vi "Dashboard Main.vi"() -> ()   [LabVIEW 2017]
uses:
  <vilib>/event_ctls.llb/eventvkey.ctl
  <vilib>/Rock Robotics/WPI/Dashboard/WPI_DashboardLogging Global.vi
  <vilib>/Utility/miscctls.llb/LVRowAndColumnTypeDef.ctl
  <vilib>/Rock Robotics/Network Tables/NT Write Numeric Array.vi
  <vilib>/Rock Robotics/Network Tables/NT Read Numeric Array.vi
panel:
  in  "Camera Settings Right":T1={"Frame Rate"=30, "Compression"=30, "Size"=1, "DB Camera Config"=FALSE} {"Frame Rate" scale=1.0..30.0; "Compression" scale=100.0..-1.0; "Size" items=["640x480", "320x240", "160x120"]}
  in  "Camera Name Right":string(combo)="No Camera Selection"
  out "Camera Info":cluster{"Mbps LED":bool, "Mbps":dbl, "fps":dbl} {"fps" format="%#.1g"; "Mbps" format="%#.1g"}
  in  "Camera Settings":T1={"Frame Rate"=30, "Compression"=30, "Size"=1, "DB Camera Config"=FALSE} {"Frame Rate" scale=1.0..30.0; "Compression" scale=100.0..-1.0; "Size" items=["640x480", "320x240", "160x120"]}
  in  "TCP":refnum<k5>
  in  "Rec Mode":enum32{"Stop", "Record", "Playback"}(radio)
  out "Robot IP":string
  out "Image Message":string="Timeout in Camera Communications"
  in  "Dashboard Tab":T2(tab)
  in  "Select Auto":string(combo)="Select Autonomous ..."
  out "NT Connection":bool
  out "MotorChart R":cluster{"Numeric":dbl, "Numeric":dbl}(graph)
  out "MotorChart L":cluster{"Numeric":dbl, "Numeric":dbl}(graph)
  out "MotorSliders R":cluster{"MotorSlide1":dbl, "MotorSlide2":dbl} {"MotorSlide2" scale=-1.0..1.0 scale format="%#_2e"; "MotorSlide1" scale=-1.0..1.0 scale format="%#_2e"}
  out "MotorSliders L":cluster{"MotorSlide1":dbl, "MotorSlide2":dbl} {"MotorSlide2" scale=-1.0..1.0 scale format="%#_2e"; "MotorSlide1" scale=-1.0..1.0 scale format="%#_2e"}
  out "Gyro":dbl(knob) scale=0.0..360.0
  out "JS1 Z":dbl(slide) scale=-1.0..1.0 scale format="%#_2e"
  out "JS1 Graph":cluster{"X":dbl, "Y":dbl}[](graph)
  out "JS1 Buttons":T3
  out "JS2 Z":dbl(slide) scale=-1.0..1.0 scale format="%#_2e"
  out "JS2 Graph":cluster{"X":dbl, "Y":dbl}[](graph)
  out "JS2 Buttons":T3
  out "Mode":T4(ring)=enum."Auto Disabled"
  out "Camera Image Right":T5(plugin-control)
  out "Left Encoder":dbl
  out "Right Encoder":dbl
  in  "Teleop Controls":T6(tab)
  in  "Y Axis":T7
  in  "X Axis":T7
  in  "Forward Trim":T8={"Trim Max"=0.37, "Trim Min"=0.01, "Trim Deadzone"=0.1, "Trim LR"=TRUE}
  in  "Backward Trim":T8={"Trim Max"=0.5, "Trim Min"=0.05, "Trim Deadzone"=0.1, "Trim LR"=FALSE}
  in  "PID Tuning":enum32{"Drive with PID", "Turn by Angle"}(tab)
  in  "Drive with PID":T9={"Max Speed"=0.7, "P/I/D"=[1.0, 0.0, 0.01], "Min Speed"=0.4, "Accel Distance"=64.0}
  in  "Turn By Angle":T10={"P/I/D"=[0.25, 0.001, 0.0], "Turn Speed"=0.55, "Linearity"=0.6}
  in  "Autonomous Distances":T11(tab)
  in  "Station 1 Angle":dbl=60.0
  in  "Station 1":dbl[](array[numeric])=[97.0, 30.0, -30.0, 120.0]
  in  "Station 2":dbl[](array[numeric])=[82.0, -48.0, 48.0, 120.0]
  in  "Station 3 Angle":dbl=-60.0
  in  "Station 3":dbl[](array[numeric])=[96.0, 30.0, -30.0, 120.0]
  in  "Drive Forward":dbl[](array[numeric])=[82.0, 0.0, 0.0, 0.0]
  in  "Gear and B":dbl[](array[numeric])=[82.0, -48.0, 0.0, 0.0]
  in  "Test Slider":dbl(slide) scale=0.0..100.0 scale format="%#_3g"
  in  "On/Off":bool caption="Solenoid"
  in  "Test Name":u16(ring) items=["Select the test to run..."]
  in  "Test Tree":string(tree)
  in  "Motor":cluster{"Value":dbl, "Enable":bool} {"Value" scale=-1.0..1.0 scale format="%#_3g"}
  out "Progress":T12 {"Test Progress" scale=0.0..100.0}
  in  "Rev/Fwd":cluster{"Forward":bool, "Reverse":bool}
  in  "Test Ring":u16(ring) items=["Monochrome", "Color"]
  out "Cmd Status":string
  in  "Execute Command":bool
  in  "Command Params":string[][](table)
  in  "Command Selection":i32(listbox)
  in  "CheckList":i32(listbox)
  out "Tree":string(tree)
  out "Camera Image":T5(plugin-control)
  in  "Camera Name":string(combo)="No Camera Selection"
  out "Background":bool
  # "HW"
  # "HW"
  # "Joysticks"
  # "Drive Motors"
  # "Front"
  # "Right"
  # "Left"
  # "Back"
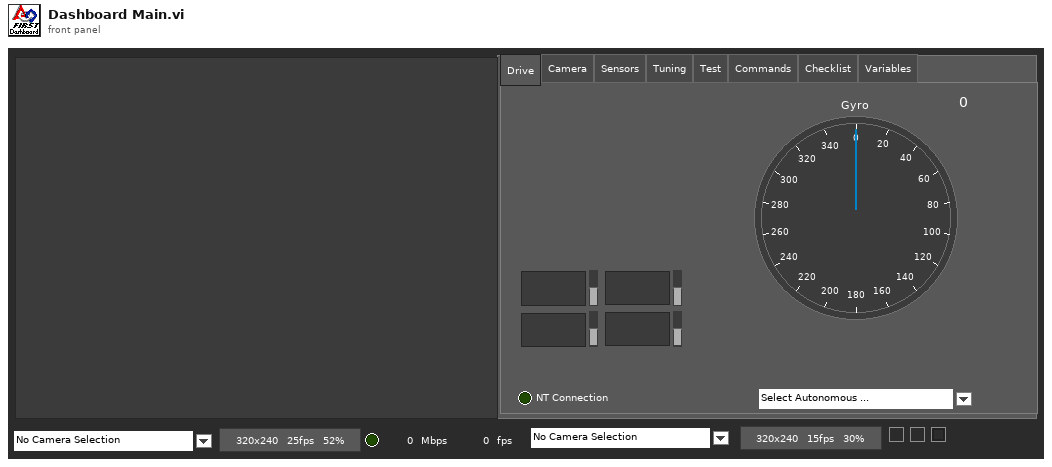
[diagram p1: front panel]
types:
  T1 = cluster{"Frame Rate":i32, "Compression":i32, "Size":u16, "DB Camera Config":bool}
  T2 = enum32{"Drive", "Camera", "Sensors", "Tuning", "Test", "Commands", "Checklist", "Variables"}
  T3 = cluster{bool, bool, bool, bool, bool, bool, bool, bool, bool, bool, bool, bool}
  T4 = enum8{"Tele-Op Disabled", "Tele-Op Enabled", "Auto Disabled", "Auto Enabled", "Test Disabled", "Test Enabled", "Disconnected", "No Code", "E-Stop"}
  T5 = typedef "IMAQ Image.ctl" = refnum<image>
  T6 = enum32{"Speed Sensitivity", "Turn Sensitivity", "Forward Trim", "Backwards Trim"}
  T7 = cluster{"Max Speed":dbl, "Min Speed":dbl, "Deadzone":dbl}
  T8 = cluster{"Trim Max":dbl, "Trim Min":dbl, "Trim Deadzone":dbl, "Trim LR":bool}
  T9 = cluster{"Max Speed":dbl, "P/I/D":dbl[], "Min Speed":dbl, "Accel Distance":dbl}
  T10 = cluster{"P/I/D":dbl[], "Turn Speed":dbl, "Linearity":dbl}
  T11 = enum32{"Station 1", "Station 2", "Station 3", "Drive Forward", "Gear and Back"}
  T12 = cluster{"Test Progress":u8, "Test Progress Text":string}
  T13 = typedef "Image Type" = u32
  T14 = cluster{"IDs":cluster{"RPC field ID":u16, "Unique ID":u16}, "String":string}
  T15 = enum32{"Drive", "Basic", "Custom", "Test", "Checklist", "Variables"}
  T16 = cluster{"Error Strings":string, "Disable Counts":cluster{u16, u16}, "Rail Faults":cluster{u16, u16, u16}, "Robot IP":string, "DB Mode":u8, "Event Info":cluster{"Name":string, "Type":u8, "Number":u16, "Replay":u8}}
  T17 = cluster{"Storage":cluster{"Disk Free":u64, "RAM Block":u32, "RAM free":u32}, "CPU Utilization":cluster{"CPU % ISR":sgl, "CPU % Time Crit":sgl, "CPU % Timed Str":sgl, "CPU % High":sgl, "CPU % Above":sgl, "CPU % Normal":sgl, "CPU % Low":sgl}, "CAN":cluster{"% Bus Utilization":sgl, "Bus Off Cnt":u32, "TX_FIFO Full Cnt":u32, "Receive Error Cnt":u8, "Transmit Error Cnt":u8}, "HID":cluster{"HID Outputs":u32, "Rumble Low":u16, "Rumble High":u16}[]}
  T18 = cluster{"Status bits":cluster{"Test Mode":bool, "Autonomous":bool, "Enabled":bool, "Code Start":bool, "Brownout":bool, "Reserved 2":bool, "Reserved 3":bool, "E-Stop":bool}, "Code Trace":cluster{"Disabled":bool, "TeleOp":bool, "Auto":bool, "Test":bool}, "Controller Type":enum16{"unknown", "cRIO", "roboRio"}, "Code?":enum16{"unknown", "noCode", "code"}, "Battery V":dbl}
  T19 = cluster{"Control Bits":cluster{"TestMode":bool, "Autonomous":bool, "Enabled":bool, "FMS Present":bool, bool, bool, bool, "E-Stop":bool}, "Team Station ":u8, "Countdown":sgl, "Joystick Values":cluster{"Axes":dbl[], "Buttons":bool[], "POVs":i16[]}[]}
  T20 = cluster{"Axes":dbl[], "Buttons":bool[], "POVs":i16[]}[]
  T21 = cluster{"Axes":dbl[], "Buttons":bool[], "POVs":i16[]}
  T22 = cluster{"Buttons[0]":bool, "Buttons[1]":bool, "Buttons[2]":bool, "Buttons[3]":bool, "Buttons[4]":bool, "Buttons[5]":bool, "Buttons[6]":bool, "Buttons[7]":bool, "Buttons[8]":bool, "Buttons[9]":bool, "Buttons[10]":bool, "Buttons[11]":bool}
  T23 = cluster{"Camera Image":refnum<vi>, "Dashboard Tab":refnum<vi>, "Background":refnum<vi>, "Rec Mode":refnum<vi>, "Test Slider":refnum<vi>, "On/Off ":refnum<vi>, "Test Ring":refnum<vi>, "Rev/Fwd":refnum<vi>, "Test Name":refnum<vi>, "Motor":refnum<vi>, "Progress":refnum<vi>, "CheckList":refnum<vi>, "Tree":refnum<vi>, "Test Tree":refnum<vi>, "Command Params":refnum<vi>, "Command Selection":refnum<vi>, "Execute Command":refnum<vi>, "Cmd Status":refnum<vi>, "Camera Settings":refnum<vi>, "Camera Name":refnum<vi>, "Camera Info":refnum<vi>, "Camera Settings Right":refnum<vi>, "Camera Name Right":refnum<vi>, "Camera Image Right":refnum<vi>}
  T24 = cluster{"Operation":enum16{"Update", "Clear"}, "Color Box":u32}[]
  T25 = typedef "eventvkey.ctl" = enum16{"ASCII", "Enter", "Return", "Shift", "Ctrl", "Alt", "Cmd", "Opt", "Caps", "NumLock", "Clear", "Break", "Up", "Down", "Left", "Right", "Insert", "Delete", "Home", "End", "PageUp", "PageDown", "Escape", "Help", "Pause", "ScrollLock", "F1", "F2", "F3", "F4", "F5", "F6", "F7", "F8", "F9", "F10", "F11", "F12", "F13", "F14", "F15", "F16", "F17", "F18", "F19", "F20", "F21", "F22", "F23", "F24", "Play", "VolumeUp", "VolumeDown", "Mute", "Two Byte Char"}
  T26 = cluster{"Image Size":bool, "Image Type":bool, "Pixel Value":bool, "ROI Information":bool, "Zoom Factor":bool}
  T27 = cluster{"Operation":enum16{"Update", "Clear"}, "Color Box":u32}
  T28 = typedef "LVRowAndColumnTypeDef.ctl" = cluster{"Row":i32, "Column":i32}
  T29 = cluster{"Shift":bool, "Ctrl":bool, "Alt":bool, "Cmd":bool, "Opt":bool}
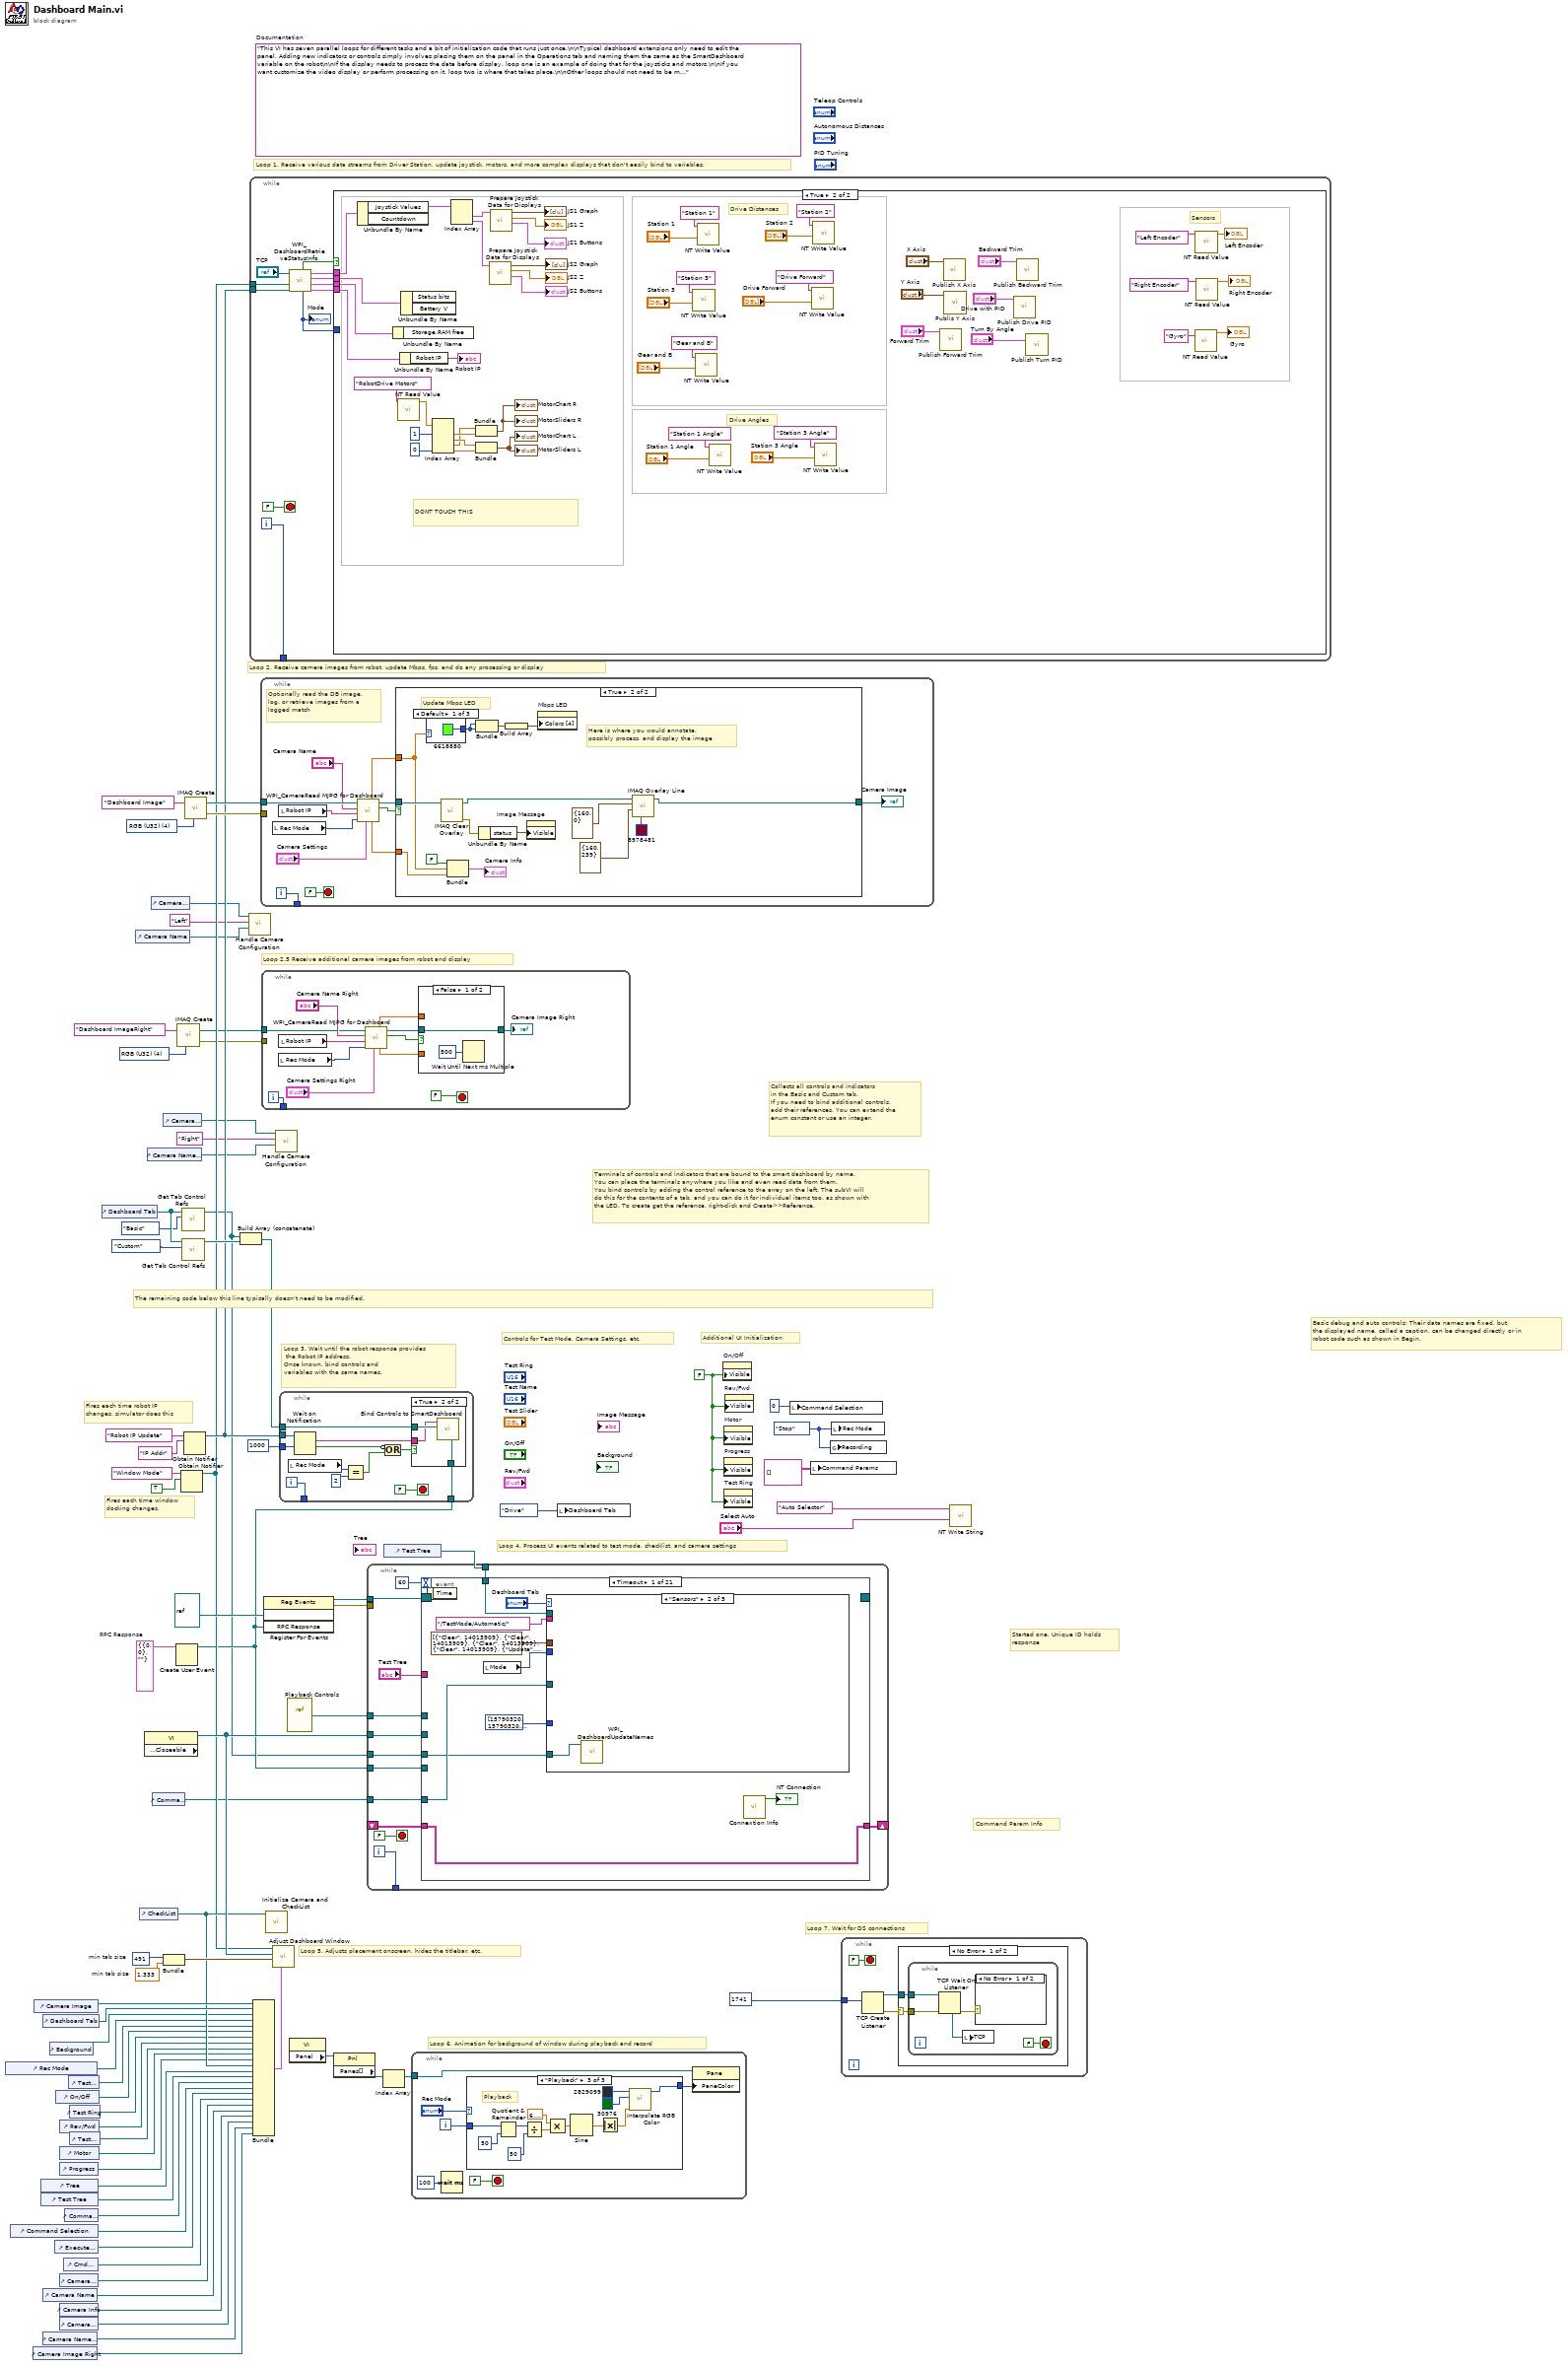
[diagram p0: block diagram]
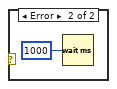
[diagram p3: hidden frame]
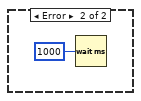
[diagram p4: hidden frame]
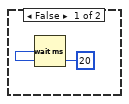
[diagram p5: hidden frame]
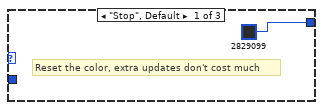
[diagram p6: hidden frame]
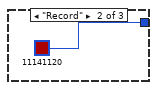
[diagram p7: hidden frame]
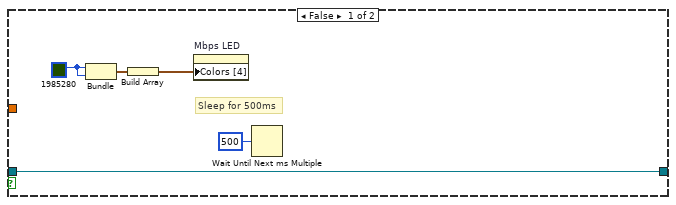
[diagram p9: hidden frame]
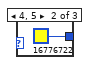
[diagram p10: hidden frame]
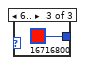
[diagram p11: hidden frame]
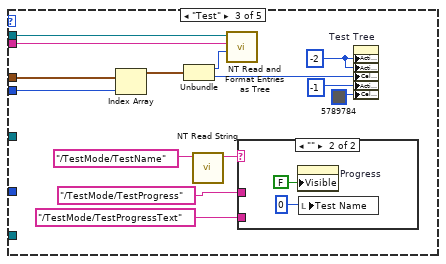
[diagram p13: hidden frame]
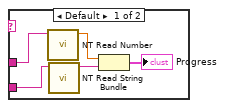
[diagram p14: hidden frame]
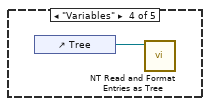
[diagram p15: hidden frame]
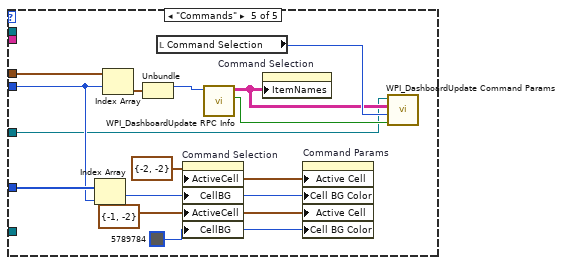
[diagram p16: hidden frame]
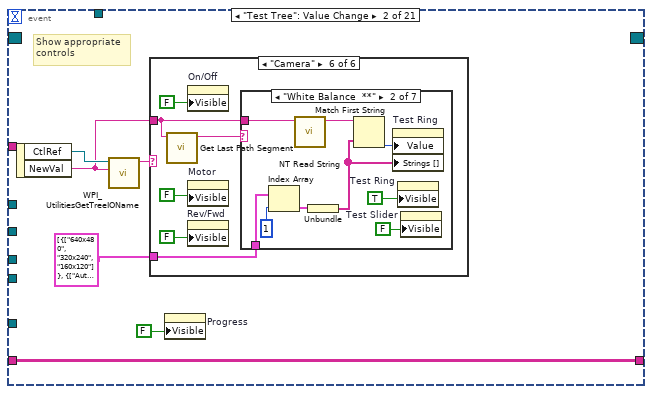
[diagram p17: hidden frame]
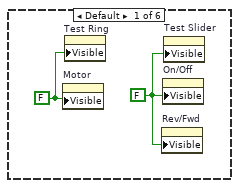
[diagram p18: hidden frame]
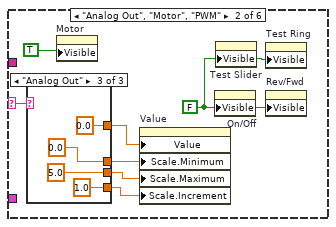
[diagram p19: hidden frame]
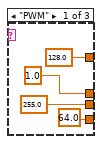
[diagram p20: hidden frame]
diagram:
  w11 = T13 4 items=["Grayscale (U8)", "Grayscale (I16)", "Grayscale (SGL)", "Complex (CSG)", "RGB (U32)", "HSL (U32)", "RGB (U64)"] ("Image Type")
  w27 = T14 {"IDs"={"RPC field ID"=0, "Unique ID"=0}, "String"=""}  # RPC Response
  w51 = 491  # min tab size
  w50 = 1.333  # min tab size
  w58 = enum32{"Stop", "Record", "Playback"}."Stop" ("Rec Mode")
  w34 = FALSE ("Visible")
  (unwired) "This VI has seven parallel loops for different tasks and a bit of initialization code that runs just once.\n\nTypical dashboard extensions only need to edit the panel. Adding new indicators or controls simply involves placing them on the panel in the Operations tab and naming them the same as the SmartDashboard variable on the robot\n\nIf the display needs to process the data before display, loop one is an example of doing that for the joysticks and motors.\n\nIf you want customize the video display or perform processing on it, loop two is where that takes place.\n\nOther loops should not need to be modified. They are pretty standard, and document the task they perform."  # Documentation
  w75 = T13 4 items=["Grayscale (U8)", "Grayscale (I16)", "Grayscale (SGL)", "Complex (CSG)", "RGB (U32)", "HSL (U32)", "RGB (U64)"] ("Image Type")
  # "Loop 2.5 Receive additional camera images from robot and display"
  # "Command Param Info"
  # "Started one, Unique ID holds\nresponse"
  # "Loop 7. Wait for DS connections"
  # "Basic debug and auto controls: Their data names are fixed, but\nthe displayed name, called a caption, can be changed directly or in\nrobot code such as shown in Begin."
  # "Controls for Test Mode, Camera Settings, etc."
  # "Additional UI Initialization"
  # "Loop 6. Animation for background of window during playback and record"
  # "Fires each time robot IP\nchanges, simulator does this"
  # "Fires each time window\ndocking changes."
  # "Collects all controls and indicators\nin the Basic and Custom tab.\nIf you need to bind additional controls,\nadd their references. You can extend the\nenum constant or use an integer."
  # "The remaining code below this line typically doesn't need to be modified."
  # "Loop 4. Process UI events related to test mode, checklist, and camera settings"
  # "Terminals of controls and indicators that are bound to the smart dashboard by name.\nYou can place the terminals anywhere you like and even read data from them.\nYou bind controls by adding the control reference to the array on the left. The subVI will\ndo this for the contents of a tab, and you can do it for individual items too, as shown with\nthe LED. To create get the reference, right-click and Create>>Reference."
  # "Loop 3. Wait until the robot response provides\n the Robot IP address.\nOnce known, bind controls and\nvariables with the same names."
  # "Loop 5. Adjusts placement onscreen, hides the titlebar, etc."
  # "Loop 1. Receive various data streams from Driver Station, update joystick, motors, and more complex displays that don't easily bind to variables."
  # "Loop 2. Receive camera images from robot, update Mbps, fps, and do any processing or display"
  n1 = control-ref of="Rec Mode"() -> (w40:refnum<vi>)
  n2 = control-ref of="Command Selection"() -> (w26:refnum<vi>)
  n3 = control-ref of="Camera Image Right"() -> (w2:refnum<vi>)
  n4 = control-ref of="Camera Image"() -> (w53:refnum<vi>)
  n5 = control-ref of="Tree"() -> (w44:refnum<vi>)
  n6 = control-ref of="Test Tree"() -> (w43:refnum<vi>)
  n7 = control-ref of="Dashboard Tab"() -> (w52:refnum<vi>)
  n8 = control-ref of="Camera Name"() -> (w17:refnum<vi>)
  n9 = control-ref of="Camera Name Right"() -> (w3:refnum<vi>)
  n10 = control-ref of="Background"() -> (w1:refnum<vi>)
  n11 = control-ref of="Execute Command"() -> (w28:refnum<vi>)
  n12 = control-ref of="On/Off"() -> (w38:refnum<vi>)
  n13 = control-ref of="Progress"() -> (w35:refnum<vi>)
  n14 = control-ref of="Camera Settings"() -> (w18:refnum<vi>)
  n15 = control-ref of="Camera Info"() -> (w16:refnum<vi>)
  n16 = control-ref of="Camera Settings Right"() -> (w4:refnum<vi>)
  n17 = control-ref of="Rev/Fwd"() -> (w36:refnum<vi>)
  n18 = control-ref of="Motor"() -> (w41:refnum<vi>)
  n19 = control-ref of="Cmd Status"() -> (w22:refnum<vi>)
  n20 = control-ref of="Command Params"() -> (w29:refnum<vi>)
  n21 = control-ref of="Test Slider"() -> (w39:refnum<vi>)
  n22 = control-ref of="Test Ring"() -> (w37:refnum<vi>)
  n23 = control-ref of="Test Name"() -> (w42:refnum<vi>)
  n24 = control-ref of="Dashboard Tab"() -> (w56:refnum<vi>)
  n25 = control-ref of="Camera Name"() -> (w19:refnum<vi>)
  n26 = control-ref of="CheckList"() -> (w45:refnum<vi>)
  n27 = property class="VI" props=["Front Panel.Closeable"]() -> (reference out=w57:refnum<vi>)  [unwired: 2 in, 2 out]
  n28 = control-ref of="Camera Name Right"() -> (w7:refnum<vi>)
  n29 = control-ref of="Camera Settings"() -> (w20:refnum<vi>)
  n30 = control-ref of="Command Params"() -> (w21:refnum<vi>)
  n31 = control-ref of="Camera Settings Right"() -> (w8:refnum<vi>)
  n32 = Bundle("min tab size"=w51, "min tab size"=w50) -> (w49:cluster{"min tab size":i32, "min tab size":dbl})  [unwired: 1 in]
  n33 = Create User Event(user event datatype=w27) -> (user event=w23:refnum<user-event>)  [unwired: 1 in, 1 out]
  n34 = call "IMAQ Create"("Image Name"="Dashboard ImageRight", "Image Type"=w11) -> ("New Image"=w10:T5, "error out"=w9:errorcluster)  [unwired: 2 in, 1 out]
  n35 = Obtain Notifier(name (unnamed)="Window Mode", notification data type=TRUE) -> (notifier out=w32:refnum<notifier>)  [unwired: 2 in, 2 out]
  n36 = call <vilib>:"Get Tab Control Refs.vi"("Page Index"=T15."Basic" ("Dashboard Tab"), "TabControl in"=w56) -> ("ControlsOnPage"=w15:refnum<vi>[])  [unwired: 9 in]
  n37 = call <vilib>:"Get Tab Control Refs.vi"("Page Index"=T15."Custom" ("Dashboard Tab"), "TabControl in"=w56) -> ("ControlsOnPage"=w55:refnum<vi>[])  [unwired: 9 in]
  n38 = Obtain Notifier(name (unnamed)="Robot IP Update", notification data type="IP Addr" ("name (unnamed)")) -> (notifier out=w33:refnum<notifier>)  [unwired: 2 in, 2 out]
  n39 = call "IMAQ Create"("Image Name"="Dashboard Image", "Image Type"=w75) -> ("New Image"=w73:T5, "error out"=w72:errorcluster)  [unwired: 2 in, 1 out]
  n40 = Build Array (concatenate)(w15, w55) -> (w54:refnum<vi>[])
  n41 = call "Handle Camera Configuration.vi"("CameraNameRef"=w19, "Camera File Name"="Left", "ClusterRef"=w20) -> ()  [unwired: 9 in]
  n42 = while {
    tunnel: [w85] -> _
    tunnel: w33 -> [w79]
    tunnel: w32 -> [w76]
    i -> [w85]
    stop <- FALSE stop-if-true
    n43 = call <vilib>:"WPI_DashboardRetrieveStatusInfo.vi"("Binding Refnum"=w79, "Window Mode Notifier"=w76, "TCP Cnx"="TCP") -> ("Power and Errors"=w80:T16, "Robot Metrics"=w83:T17, "Status Info"=w84:T18, "Control Info"=w81:T19, "Robot Mode"=w78:T4, "Process?"=w82:bool)  [unwired: 3 in]
    "Mode" <- w78
    n44 = case shown="True" w82 {
      tunnel: w84 -> [_ w137]
      tunnel: w83 -> [_ w136]
      tunnel: w81 -> [_ w135]
      tunnel: w80 -> [_ w134]
      tunnel: w78 -> [_ _]
      frame False {
        n45 = Wait (ms)(milliseconds to wait=u32 20) -> ()  [unwired: 1 out]
      }
      frame True {
        # "Drive Angles"
        # "Sensors"
        # "Drive Distances"
        # "DONT TOUCH THIS"
        n46 = Unbundle By Name(w135) -> ("Joystick Values"=w125:T20)  [unwired: 1 out]
        n47 = Unbundle By Name(w136) -> ()  [unwired: 1 out]
        n48 = call-poly <vilib>:"NT Read Value.vi"("Name"="RobotDrive Motors") -> ("Numeric Array"=w115:dbl[])  [unwired: 9 in, 1 out]
        n49 = Unbundle By Name(w134) -> ("Robot IP"=→"Robot IP":string)
        n50 = Unbundle By Name(w137) -> ()  [unwired: 2 out]
        n51 = Index Array(array=w115, index #1=1, index #4=0) -> (element #1=w129:dbl, element #2=w130:dbl, element #3=w128:dbl, element #4=w133:dbl)  [unwired: 2 in]
        n52 = Index Array(array=w125) -> (element #1=w124:T21, element #2=w120:T21)  [unwired: 2 in]
        n53 = Bundle("Numeric"=w128, "Numeric"=w129) -> (→"MotorChart R" →"MotorSliders R":cluster{"Numeric":dbl, "Numeric":dbl})  [unwired: 1 in]
        n54 = Bundle("Numeric"=w130, "Numeric"=w133) -> (→"MotorChart L" →"MotorSliders L":cluster{"Numeric":dbl, "Numeric":dbl})  [unwired: 1 in]
        n55 = call "Prepare Joystick Data for Displays.vi"("Joystick Values"=w120) -> ("Buttons"=→"JS2 Buttons":T22, "Z Axis"=→"JS2 Z":dbl, "Cartesian Data"=→"JS2 Graph":cluster{"X axis":dbl, "X axis":dbl}[])  [unwired: 8 in]
        n56 = call "Prepare Joystick Data for Displays.vi"("Joystick Values"=w124) -> ("Buttons"=→"JS1 Buttons":T22, "Z Axis"=→"JS1 Z":dbl, "Cartesian Data"=→"JS1 Graph":cluster{"X axis":dbl, "X axis":dbl}[])  [unwired: 8 in]
        n57 = call-poly <vilib>:"NT Write Value.vi"("Numeric Array"="Station 3", "Name"="Station 3") -> ()  [unwired: 9 in, 1 out]
        n58 = call-poly <vilib>:"NT Write Value.vi"("Numeric Array"="Gear and B", "Name"="Gear and B") -> ()  [unwired: 9 in, 1 out]
        n59 = call-poly <vilib>:"NT Write Value.vi"("Numeric Array"="Station 1", "Name"="Station 1") -> ()  [unwired: 9 in, 1 out]
        n60 = call-poly <vilib>:"NT Write Value.vi"("Numeric"="Station 1 Angle", "Name"="Station 1 Angle") -> ()  [unwired: 9 in, 1 out]
        n61 = call-poly <vilib>:"NT Write Value.vi"("Numeric Array"="Drive Forward", "Name"="Drive Forward") -> ()  [unwired: 9 in, 1 out]
        n62 = call-poly <vilib>:"NT Write Value.vi"("Numeric Array"="Station 2", "Name"="Station 2") -> ()  [unwired: 9 in, 1 out]
        n63 = call-poly <vilib>:"NT Write Value.vi"("Numeric"="Station 3 Angle", "Name"="Station 3 Angle") -> ()  [unwired: 9 in, 1 out]
        n64 = call "Publish Forward Trim.vi"("Forward Trim"="Forward Trim") -> ()  [unwired: 11 in]
        n65 = call "Publish X Axis.vi"("X Axis"="X Axis") -> ()  [unwired: 11 in]
        n66 = call "Publis Y Axis.vi"("Y Axis"="Y Axis") -> ()  [unwired: 11 in]
        n67 = call "Publish Drive PID.vi"("Drive with PID"="Drive with PID") -> ()  [unwired: 11 in]
        n68 = call "Publish Backward Trim.vi"("Backward Trim"="Backward Trim") -> ()  [unwired: 11 in]
        n69 = call "Publish Turn PID.vi"("Turn By Angle"="Turn By Angle") -> ()  [unwired: 11 in]
        n70 = call-poly <vilib>:"NT Read Value.vi"("Name"="Gyro") -> ("Numeric"=→"Gyro":dbl)  [unwired: 9 in, 1 out]
        n71 = call-poly <vilib>:"NT Read Value.vi"("Name"="Left Encoder") -> ("Numeric"=→"Left Encoder":dbl)  [unwired: 9 in, 1 out]
        n72 = call-poly <vilib>:"NT Read Value.vi"("Name"="Right Encoder") -> ("Numeric"=→"Right Encoder":dbl)  [unwired: 9 in, 1 out]
      }
    }
  }
  n73 = Bundle("Camera Image"=w53, "Dashboard Tab"=w52, "Background"=w1, "Rec Mode"=w40, "Test Slider"=w39, "On/Off"=w38, "Test Ring"=w37, "Rev/Fwd"=w36, "Test Name"=w42, "Motor"=w41, "Progress"=w35, "CheckList"=w45, "Tree"=w44, "Test Tree"=w43, "Command Params"=w29, "Command Selection"=w26, "Execute Command"=w28, "Cmd Status"=w22, "Camera Settings"=w18, "Camera Name"=w17, "Camera Info"=w16, "Camera Settings Right"=w4, "Camera Name Right"=w3, "Camera Image Right"=w2) -> (w46:T23)  [unwired: 1 in]
  n74 = while {
    tunnel: w73 -> [w147]
    tunnel: w72 -> [_]
    tunnel: [w148] -> _
    i -> [w148]
    stop <- FALSE stop-if-true
    # "Optionally read the DB image,\nlog, or retrieve images from a\nlogged match"
    n75 = local read "Rec Mode"() -> (w143:enum32{"Stop", "Record", "Playback"})
    n76 = local read "Robot IP"() -> (w142:string)
    n77 = call <vilib>:"WPI_CameraRead MJPG for Dashboard.vi"("Camera Settings"="Camera Settings", "Rec Mode"=w143, "NT Connection"=w142, "Capture Info"="Camera Name", "Refnum in"=w147) -> ("Active"=w145:bool, "Refnum out"=w146:T5, "FPS"=w144:dbl, "Bandwidth (Mbps)"=w141:dbl)  [unwired: 3 in]
    n78 = case shown="True" w145 {
      tunnel: w146 -> [w150 w165]
      tunnel: w141 -> [_ w162]
      tunnel: w144 -> [_ w163]
      tunnel: [w150 w158] -> w138
      frame False {
        w152 = u32 1985280 ("Color Box")
        # "Sleep for 500ms"
        n79 = Bundle("Color Box"=w152, "Color Box"=w152) -> (w153:cluster{"Color Box":u32, "Color Box":u32})  [unwired: 1 out]
        n80 = Build Array(w153) -> (w151:cluster{"Color Box":u32, "Color Box":u32}[])
        n81 = property on="Mbps LED" class="Bool (strict)"("Colors [4]"=w151) -> ()  [unwired: 2 in, 2 out]
        n82 = Wait Until Next ms Multiple(millisecond multiple=u32 500) -> ()  [unwired: 1 out]
      }
      frame True {
        # "Here is where you would annotate,\npossibly process, and display the image"
        # "Update Mbps LED"
        n83 = case shown="Default" w162 {
          tunnel: [u32 6618880 ("Color Box") u32 16776722 ("Color Box") u32 16716800 ("Color Box")] -> w166
          frame Default {
          }
          frame 4, 5 {
          }
          frame 6.. {
          }
        }
        n84 = call "IMAQ Clear Overlay"("Image"=w165) -> ("error out"=w168:errorcluster, "Image Out"=w159:T5)  [unwired: 2 in, 7 out]
        n85 = Bundle(FALSE, "Bandwidth (Mbps)"=w162, "FPS"=w163) -> (→"Camera Info":cluster{bool, "Bandwidth (Mbps)":dbl, "FPS":dbl})  [unwired: 1 in]
        n86 = Bundle("Color Box"=w166, "Color Box"=w166) -> (w167:cluster{"Color Box":u32, "Color Box":u32})  [unwired: 1 out]
        n87 = Unbundle By Name(w168) -> ("status"=w169:bool)
        n88 = Build Array(w167) -> (w164:cluster{"Color Box":u32, "Color Box":u32}[])
        n89 = property on="Image Message" class="Str"("Visible"=w169) -> ()  [unwired: 2 in, 2 out]
        n90 = property on="Mbps LED" class="Bool (strict)"("Colors [4]"=w164) -> ()  [unwired: 2 in, 2 out]
        n91 = call "IMAQ Overlay Line"("Color"=u32 8978481, "End Point"=cluster{"X":i32, "Y":i32} {"X"=160, "Y"=239}, "Start Point"=cluster{"X":i32, "Y":i32} {"X"=160, "Y"=0}, "Image"=w159) -> ("Image Out"=w158:T5)  [unwired: 6 in, 1 out]
      }
    }
    "Camera Image" <- w138
  }
  n92 = while {
    tunnel: w10 -> [w183]
    tunnel: w9 -> [_]
    tunnel: [w177] -> _
    i -> [w177]
    stop <- FALSE stop-if-true
    n93 = local read "Rec Mode"() -> (w181:enum32{"Stop", "Record", "Playback"})
    n94 = local read "Robot IP"() -> (w182:string)
    n95 = call <vilib>:"WPI_CameraRead MJPG for Dashboard.vi"("Camera Settings"="Camera Settings Right", "Rec Mode"=w181, "NT Connection"=w182, "Capture Info"="Camera Name Right", "Refnum in"=w183) -> ("Active"=w176:bool, "Refnum out"=w179:T5, "FPS"=w174:dbl, "Bandwidth (Mbps)"=w175:dbl)  [unwired: 3 in]
    n96 = case shown="False" w176 {
      tunnel: w179 -> [w185 w187]
      tunnel: w175 -> [_ _]
      tunnel: w174 -> [_ _]
      tunnel: [w185 w187] -> w173
      frame False {
        n97 = Wait Until Next ms Multiple(millisecond multiple=u32 500) -> ()  [unwired: 1 out]
      }
      frame True {
      }
    }
    "Camera Image Right" <- w173
  }
  n98 = register-events(refnum<vi> refnum, w23) -> (reference out=w62:refnum<event-registration>, error out=w61:errorcluster)  [unwired: 2 in]
  n99 = call "Initialize Camera and CheckList.vi"("ListBox in"=w45) -> ()  [unwired: 11 in]
  n100 = call "Adjust Dashboard Window.vi"("Sizing Refnums"=w46, "Size Constraints"=w49, "VI"=w57, "WIn Mode"=w32) -> ()  [unwired: 8 in]
  n101 = call "Handle Camera Configuration.vi"("CameraNameRef"=w7, "Camera File Name"="Right", "ClusterRef"=w8) -> ()  [unwired: 9 in]
  n102 = while {
    tunnel: w54 -> [w199]
    tunnel: w33 -> [w197]
    tunnel: [w195] -> _
    tunnel: u32 1000 ("milliseconds to wait") -> [w194]
    tunnel: w23 -> [w188]
    i -> [w195]
    stop <- FALSE stop-if-true
    n103 = local read "Rec Mode"() -> (w190:enum32{"Stop", "Record", "Playback"})
    n104 = Wait on Notification(notifier=w197, timeout in ms (-1)=w194) -> (notification=w196:string, timed out?=w192:bool)  [unwired: 2 in, 2 out]
    n105 = Equal?(x=w190, y=u16 2 ("Rec Mode")) -> (x = y?=w191:bool)
    n106 = Compound Arithmetic op=OR(invert w192, w191) -> (w193:bool)
    n107 = case shown="True" w193 {
      tunnel: w199 -> [_ w202]
      tunnel: w196 -> [_ w201]
      tunnel: w188 -> [_ w200]
      frame False {
      }
      frame True {
        n108 = call <vilib>:"Bind Controls to SmartDashboard.vi"("RPC ref"=w200, "Bound Control Refs"=w202, "Server IP Address"=w201) -> ()  [unwired: 9 in]
      }
    }
  }
  n109 = vi-ref "Playback Controls.vi"() -> (w63:refnum<vi>)
  n110 = property class="VI"() -> ("Panel"=w65:refnum<vi>)  [unwired: 2 in, 2 out]
  n111 = property class="Pnl"(reference=w65) -> ("Panes[]"=w66:refnum<vi>[])  [unwired: 1 in, 2 out]
  n112 = Index Array(array=w66) -> (element=w64:refnum<vi>)  [unwired: 1 in]
  n113 = control-ref of="Test Tree"() -> (w67:refnum<vi>)
  n114 = while {
    tunnel: [w212] -> _
    tunnel: w67 -> [w211]
    tunnel: w63 -> [w210]
    tunnel: w62 -> [w209]
    tunnel: w61 -> [_]
    tunnel: w57 -> [w208]
    tunnel: w23 -> [w207]
    tunnel: w21 -> [w206]
    shift-right: [w205] -> _
    shift-left: _ -> [w204]
    tunnel: w15 -> [w203]
    i -> [w212]
    stop <- FALSE stop-if-true
    n115 = event shown="[0] Timeout" {
      selector: w209 -> [_ _ _ _ _ _ _ _ _ _ _ _ _ _ _ _ _ _ _ _ _]
      dyn-events: [_ _ _ _ _ _ _ _ _ _ _ _ _ _ _ _ w468 _ _ _ _] -> _
      timeout: u32 60 ("milliseconds to wait") -> [_ _ _ _ _ _ _ _ _ _ _ _ _ _ _ _ _ _ _ _ _]
      tunnel: w211 -> [w224 _ _ _ _ _ _ _ _ _ _ _ _ _ _ _ _ _ _ _ _]
      tunnel: "Test Tree" -> [_ _ _ _ _ _ _ _ _ _ _ w435 w443 w445 w449 w457 _ _ _ _ _]
      tunnel: w210 -> [_ _ _ _ _ _ _ _ _ _ _ _ _ _ _ _ w470 _ w488 _ _]
      tunnel: w208 -> [_ _ _ _ _ _ _ _ _ _ _ _ _ _ _ _ w466 _ _ _ _]
      tunnel: w207 -> [_ _ _ _ _ _ _ _ _ _ _ _ _ _ _ _ w462 _ _ _ _]
      tunnel: w206 -> [w219 _ _ _ _ _ w386 _ _ _ _ _ _ _ _ _ _ _ _ _ _]
      tunnel: [w218 w263 w365 w370 w379 w383 w384 w393 w403 w410 w422 w434 w441 w444 w448 w456 w461 w483 w485 w489 w500] -> w205
      tunnel: w204 -> [w218 w263 w365 w370 w379 w383 w384 _ _ w410 w422 w434 w441 w444 w448 w456 w461 w483 w485 w489 w500]
      tunnel: w203 -> [w216 _ _ _ _ _ _ _ _ _ _ _ _ _ _ _ _ _ _ _ _]
      event Timeout {
        n116 = event-data() -> ()  [unwired: 1 in, 1 out]
        n117 = local read "Mode"() -> (w221:T4)
        n118 = case shown="\"Sensors\"" "Dashboard Tab" {
          tunnel: w224 -> [_ _ w240 _ _]
          tunnel: "/TestMode/Automatic/" ("Name Pattern") -> [_ _ w239 _ _]
          tunnel: T24 [{"Operation"=enum."Clear", "Color Box"=14013909}, {"Operation"=enum."Clear", "Color Box"=14013909}, {"Operation"=enum."Clear", "Color Box"=14013909}, {"Operation"=enum."Clear", "Color Box"=14013909}, {"Operation"=enum."Update", "Color Box"=14013909}, {"Operation"=enum."Update", "Color Box"=16777215}, {"Operation"=enum."Clear", "Color Box"=14013909}, {"Operation"=enum."Clear", "Color Box"=14013909}, {"Operation"=enum."Clear", "Color Box"=14013909}] -> [_ _ w232 _ w256]
          tunnel: w221 -> [_ _ w231 _ w255]
          tunnel: u32[] [15790320, 15790320, 15790320, 15790320, 16777215, 16777215, 15790320, 15790320, 15790320] -> [_ _ _ _ w261]
          tunnel: w219 -> [_ _ _ _ w249]
          tunnel: w216 -> [_ w226 _ _ _]
          frame "Tuning", Default {
          }
          frame "Sensors" {
            n119 = call <vilib>:"WPI_DashboardUpdateNames.vi"("Controls on Tab"=w226) -> ()  [unwired: 11 in]
          }
          frame "Test" {
            w238 = -2 ("Active Item:Row Number")
            n120 = Index Array(array=w232, index=w231) -> (element=w233:T27)
            n121 = Unbundle(w233) -> ("Operation"=w234:enum16{"Update", "Clear"}, "Color Box"=w235:u32)
            n122 = call <vilib>:"NT Read String.vi"("Name"="/TestMode/TestName") -> ("String"=w229:string)  [unwired: 9 in, 1 out]
            n123 = call <vilib>:"NT Read and Format Entries as Tree.vi"("Operation"=w234, "Name Pattern"=w239, "Tree Refnum"=w240) -> ()  [unwired: 7 in, 2 out]
            n124 = case shown="\"\"" w229 {
              tunnel: "/TestMode/TestProgress" ("Name") -> [w242 _]
              tunnel: "/TestMode/TestProgressText" ("Name") -> [w241 _]
              frame Default {
                n125 = call <vilib>:"NT Read Number.vi"("Name"=w242) -> ("Numeric"=w243:dbl)  [unwired: 9 in, 1 out]
                n126 = call <vilib>:"NT Read String.vi"("Name"=w241) -> ("String"=w244:string)  [unwired: 9 in, 1 out]
                n127 = Bundle("Numeric"=w243, "String"=w244) -> (→"Progress":cluster{"Numeric":dbl, "String":string})  [unwired: 1 in]
              }
              frame "" {
                n128 = property on="Progress" class="Clust (strict)"("Visible"=FALSE) -> ()  [unwired: 2 in, 2 out]
                n129 = local write "Test Name"(u16 0) -> ()
              }
            }
            n130 = property on="Test Tree" class="Tree (strict)"("Active Item Row Number"=w238, "ActiveColNum"=w238, "CellBG"=w235, "Active Item Row Number"=-1 ("Active Item:Row Number"), "CellBG"=u32 5789784 ("Color Box")) -> ()  [unwired: 2 in, 2 out]
          }
          frame "Variables" {
            n131 = control-ref of="Tree"() -> (w248:refnum<vi>)
            n132 = call <vilib>:"NT Read and Format Entries as Tree.vi"("Tree Refnum"=w248) -> ()  [unwired: 9 in, 2 out]
          }
          frame "Commands" {
            w257 = u32 5789784 ("Color Box")
            w258 = T28 {"Row"=-1, "Column"=-2} ("Active Cell:Active Cell")
            w260 = T28 {"Row"=-2, "Column"=-2} ("Active Cell:Active Cell")
            n133 = Index Array(array=w261, index=w255) -> (element=w259:u32)
            n134 = Index Array(array=w256, index=w255) -> (element=w254:T27)
            n135 = Unbundle(w254) -> ("Operation"=w253:enum16{"Update", "Clear"})  [unwired: 1 out]
            n136 = local read "Command Selection"() -> (w252:i32)
            n137 = property on="Command Selection" class="MCListbox (strict)"("ActiveCell"=w260, "CellBG"=w259, "ActiveCell"=w258, "CellBG"=w257) -> ()  [unwired: 2 in, 2 out]
            n138 = call <vilib>:"WPI_DashboardUpdate RPC Info.vi"("Operation"=w253) -> ("update"=w251:bool, "commands"=w250:string[][])  [unwired: 9 in]
            n139 = property on="Command Selection" class="MCListbox (strict)"("ItemNames"=w250) -> ()  [unwired: 2 in, 2 out]
            n140 = property on="Command Params" class="Tbl (strict)"("Active Cell"=w260, "Cell BG Color"=w259, "Active Cell"=w258, "Cell BG Color"=w257) -> ()  [unwired: 2 in, 2 out]
            n141 = call <vilib>:"WPI_DashboardUpdate Command Params.vi"("Update"=w251, "NewVal"=w252, "Commands"=w250, "Param Tbl"=w249) -> ()  [unwired: 7 in, 1 out]
          }
        }
        n142 = call <vilib>:"Connextion Info.vi"() -> ("Connected"=→"NT Connection":bool)  [unwired: 10 in, 1 out]
      }
      event "Test Tree": Value Change {
        # "Show appropriate\ncontrols"
        n143 = event-data() -> ("CtlRef"=w266:refnum<vi>, "NewVal"=w264:string)  [unwired: 1 in]
        n144 = call <vilib>:"WPI_UtilitiesGetTreeIOName.vi"("NewVal"=w264, "TreeControl in"=w266) -> ("I/O Name"=w267:string)  [unwired: 9 in]
        n145 = case shown="\"Camera\"" w267 {
          selector: w267 -> [_ w274 _ w296 w305 _]
          tunnel: w264 -> [_ _ w293 w295 _ w312]
          tunnel: cluster{string[]}[] [{["640x480", "320x240", "160x120"]}, {["Auto", "Fixed indoor", "Fixed outdoor 1", "Fixed outdoor 2", "Fixed fluorescent 1", "Fixed fluorescent 2", "Hold current"]}, {["Auto", "Flicker-free 50 Hz", "Flicker-free 60 Hz", "Hold current"]}, {["None", "Prioritize frame rate", "Prioritize image quality"]}, {["Monochrome", "Color"]}] -> [_ _ _ _ _ w311]
          frame Default {
            w269 = FALSE ("Visible")
            w268 = FALSE ("Visible")
            n146 = property on="Motor" class="Clust (strict)"("Visible"=w268) -> ()  [unwired: 2 in, 2 out]
            n147 = property on="Test Ring" class="Ring (strict)"("Visible"=w268) -> ()  [unwired: 2 in, 2 out]
            n148 = property on="Rev/Fwd" class="Clust (strict)"("Visible"=w269) -> ()  [unwired: 2 in, 2 out]
            n149 = property on="On/Off" class="Bool (strict)"("Visible"=w269) -> ()  [unwired: 2 in, 2 out]
            n150 = property on="Test Slider" class="Slide (strict)"("Visible"=w269) -> ()  [unwired: 2 in, 2 out]
          }
          frame "Analog Out", "Motor", "PWM" {
            w275 = FALSE ("Visible")
            n151 = case shown="\"Analog Out\"" w274 {
              tunnel: [1.0 ("Value") -1.0 ("Value") 0.0 ("Value")] -> w273
              tunnel: [255.0 ("Value") 1.0 ("Value") 5.0 ("Value")] -> w272
              tunnel: [128.0 ("Value") 0.0 ("Value") 0.0 ("Value")] -> w271
              tunnel: [64.0 ("Value") 0.5 ("Value") 1.0 ("Value")] -> w270
              frame "PWM" {
              }
              frame "Motor", Default {
              }
              frame "Analog Out" {
              }
            }
            n152 = property on="Motor" class="Clust (strict)"("Visible"=TRUE) -> ()  [unwired: 2 in, 2 out]
            n153 = property on="Value" class="Slide (strict)"("Value"=w271, "Scale.Minimum"=w273, "Scale.Maximum"=w272, "Scale.Increment"=w270) -> ()  [unwired: 2 in, 2 out]
            n154 = property on="On/Off" class="Bool (strict)"("Visible"=w275) -> ()  [unwired: 2 in, 2 out]
            n155 = property on="Test Slider" class="Slide (strict)"("Visible"=w275) -> ()  [unwired: 2 in, 2 out]
            n156 = property on="Test Ring" class="Ring (strict)"("Visible"=w275) -> ()  [unwired: 2 in, 2 out]
            n157 = property on="Rev/Fwd" class="Clust (strict)"("Visible"=w275) -> ()  [unwired: 2 in, 2 out]
          }
          frame "Servo" {
            w291 = FALSE ("Visible")
            n158 = call <vilib>:"NT Read Number.vi"("Name"=w293) -> ("Numeric"=w292:dbl)  [unwired: 9 in, 1 out]
            n159 = property on="Test Slider" class="Slide (strict)"("Visible"=TRUE, "Scale.Maximum"=170.0 ("Scale.Range:Maximum")) -> ()  [unwired: 2 in, 2 out]
            n160 = local write "Test Slider"(w292) -> ()
            n161 = property on="Motor" class="Clust (strict)"("Visible"=w291) -> ()  [unwired: 2 in, 2 out]
            n162 = property on="Rev/Fwd" class="Clust (strict)"("Visible"=w291) -> ()  [unwired: 2 in, 2 out]
            n163 = property on="On/Off" class="Bool (strict)"("Visible"=w291) -> ()  [unwired: 2 in, 2 out]
            n164 = property on="Test Ring" class="Ring (strict)"("Visible"=w291) -> ()  [unwired: 2 in, 2 out]
          }
          frame "Relay", "Solenoid" {
            w294 = FALSE ("Visible")
            n165 = property on="Motor" class="Clust (strict)"("Visible"=w294) -> ()  [unwired: 2 in, 2 out]
            n166 = property on="Test Slider" class="Slide (strict)"("Visible"=w294) -> ()  [unwired: 2 in, 2 out]
            n167 = Search and Replace String(input string=w295, search string="/Value  **", replace string="/Direction") -> (result string=w301:string)  [unwired: 5 in, 3 out]
            n168 = property on="Test Ring" class="Ring (strict)"("Visible"=w294) -> ()  [unwired: 2 in, 2 out]
            n169 = call <vilib>:"NT Read String.vi"("Name"=w301) -> ("String"=w299:string)  [unwired: 9 in, 1 out]
            n170 = Equal?(x="Both directions", y=w299) -> (x = y?=w297:bool)
            n171 = Not(x=w297) -> (.not. x?=w298:bool)
            n172 = property on="Rev/Fwd" class="Clust (strict)"("Visible"=w297) -> ()  [unwired: 2 in, 2 out]
            n173 = property on="On/Off" class="Bool (strict)"("Visible"=w298, "Caption.Text"=w296) -> ()  [unwired: 2 in, 2 out]
          }
          frame "Compressor", "Digital Out" {
            w304 = FALSE ("Visible")
            # "Get direction and finish"
            n174 = property on="Motor" class="Clust (strict)"("Visible"=w304) -> ()  [unwired: 2 in, 2 out]
            n175 = property on="Test Slider" class="Slide (strict)"("Visible"=w304) -> ()  [unwired: 2 in, 2 out]
            n176 = property on="Test Ring" class="Ring (strict)"("Visible"=w304) -> ()  [unwired: 2 in, 2 out]
            n177 = property on="On/Off" class="Bool (strict)"("Visible"=TRUE, "Caption.Text"=w305) -> ()  [unwired: 2 in, 2 out]
            n178 = property on="Rev/Fwd" class="Clust (strict)"("Visible"=FALSE) -> ()  [unwired: 2 in, 2 out]
          }
          frame "Camera" {
            n179 = call <vilib>:"Get Last Path Segment.vi"("String in"=w312) -> ("String out"=w313:string)  [unwired: 10 in]
            n180 = property on="On/Off" class="Bool (strict)"("Visible"=FALSE) -> ()  [unwired: 2 in, 2 out]
            n181 = property on="Motor" class="Clust (strict)"("Visible"=FALSE) -> ()  [unwired: 2 in, 2 out]
            n182 = property on="Rev/Fwd" class="Clust (strict)"("Visible"=FALSE) -> ()  [unwired: 2 in, 2 out]
            n183 = case shown="\"White Balance  **\"" w313 {
              tunnel: w312 -> [w319 w328 w337 w346 w355 _ w361]
              tunnel: w311 -> [w317 w325 w334 w343 w352 _ _]
              frame "Size  **" {
                n184 = Index Array(array=w317) -> (element=w316:cluster{string[]})  [unwired: 1 in]
                n185 = call <vilib>:"NT Read String.vi"("Name"=w319) -> ("String"=w318:string)  [unwired: 9 in, 1 out]
                n186 = Unbundle(w316) -> (w314:string[])
                n187 = Match First String(2:w314, 3:w318) -> (0:w315:i32)  [unwired: 1 out]
                n188 = property on="Test Ring" class="Ring (strict)"("Value"=w315, "Strings []"=w314) -> ()  [unwired: 2 in, 2 out]
                n189 = property on="Test Ring" class="Ring (strict)"("Visible"=TRUE) -> ()  [unwired: 2 in, 2 out]
                n190 = property on="Test Slider" class="Slide (strict)"("Visible"=FALSE) -> ()  [unwired: 2 in, 2 out]
              }
              frame "White Balance  **" {
                n191 = Index Array(array=w325, index=1) -> (element=w326:cluster{string[]})
                n192 = call <vilib>:"NT Read String.vi"("Name"=w328) -> ("String"=w327:string)  [unwired: 9 in, 1 out]
                n193 = Unbundle(w326) -> (w323:string[])
                n194 = Match First String(2:w323, 3:w327) -> (0:w322:i32)  [unwired: 1 out]
                n195 = property on="Test Ring" class="Ring (strict)"("Value"=w322, "Strings []"=w323) -> ()  [unwired: 2 in, 2 out]
                n196 = property on="Test Ring" class="Ring (strict)"("Visible"=TRUE) -> ()  [unwired: 2 in, 2 out]
                n197 = property on="Test Slider" class="Slide (strict)"("Visible"=FALSE) -> ()  [unwired: 2 in, 2 out]
              }
              frame "Exposure  **" {
                n198 = Index Array(array=w334, index=2) -> (element=w335:cluster{string[]})
                n199 = call <vilib>:"NT Read String.vi"("Name"=w337) -> ("String"=w336:string)  [unwired: 9 in, 1 out]
                n200 = Unbundle(w335) -> (w331:string[])
                n201 = Match First String(2:w331, 3:w336) -> (0:w332:i32)  [unwired: 1 out]
                n202 = property on="Test Ring" class="Ring (strict)"("Value"=w332, "Strings []"=w331) -> ()  [unwired: 2 in, 2 out]
                n203 = property on="Test Ring" class="Ring (strict)"("Visible"=TRUE) -> ()  [unwired: 2 in, 2 out]
                n204 = property on="Test Slider" class="Slide (strict)"("Visible"=FALSE) -> ()  [unwired: 2 in, 2 out]
              }
              frame "Exposure Priority  **" {
                n205 = Index Array(array=w343, index=3) -> (element=w344:cluster{string[]})
                n206 = call <vilib>:"NT Read String.vi"("Name"=w346) -> ("String"=w345:string)  [unwired: 9 in, 1 out]
                n207 = Unbundle(w344) -> (w340:string[])
                n208 = Match First String(2:w340, 3:w345) -> (0:w341:i32)  [unwired: 1 out]
                n209 = property on="Test Ring" class="Ring (strict)"("Value"=w341, "Strings []"=w340) -> ()  [unwired: 2 in, 2 out]
                n210 = property on="Test Ring" class="Ring (strict)"("Visible"=TRUE) -> ()  [unwired: 2 in, 2 out]
                n211 = property on="Test Slider" class="Slide (strict)"("Visible"=FALSE) -> ()  [unwired: 2 in, 2 out]
              }
              frame "Color Enable  **" {
                n212 = Index Array(array=w352, index=4) -> (element=w353:cluster{string[]})
                n213 = call <vilib>:"NT Read String.vi"("Name"=w355) -> ("String"=w354:string)  [unwired: 9 in, 1 out]
                n214 = Unbundle(w353) -> (w349:string[])
                n215 = Match First String(2:w349, 3:w354) -> (0:w350:i32)  [unwired: 1 out]
                n216 = property on="Test Ring" class="Ring (strict)"("Value"=w350, "Strings []"=w349) -> ()  [unwired: 2 in, 2 out]
                n217 = property on="Test Ring" class="Ring (strict)"("Visible"=TRUE) -> ()  [unwired: 2 in, 2 out]
                n218 = property on="Test Slider" class="Slide (strict)"("Visible"=FALSE) -> ()  [unwired: 2 in, 2 out]
              }
              frame Default {
                n219 = property on="Test Ring" class="Ring (strict)"("Visible"=FALSE) -> ()  [unwired: 2 in, 2 out]
                n220 = property on="Test Slider" class="Slide (strict)"("Visible"=FALSE) -> ()  [unwired: 2 in, 2 out]
              }
              frame "Brightness  **", "Color Level  **", "Compression  **", "FPS  **", "Sharpness  **" {
                n221 = call <vilib>:"NT Read Number.vi"("Name"=w361) -> ("Numeric"=w360:dbl)  [unwired: 9 in, 1 out]
                n222 = local write "Test Slider"(w360) -> ()
                n223 = property on="Test Slider" class="Slide (strict)"("Visible"=TRUE, "Scale.Maximum"=100.0 ("Scale.Range:Maximum")) -> ()  [unwired: 2 in, 2 out]
                n224 = property on="Test Ring" class="Ring (strict)"("Visible"=FALSE) -> ()  [unwired: 2 in, 2 out]
              }
            }
          }
        }
        n225 = property on="Progress" class="Clust (strict)"("Visible"=FALSE) -> ()  [unwired: 2 in, 2 out]
      }
      event "Test Name": Mouse Enter {
        # "Populate the ring with the list of tests"
        n226 = event-data() -> ()  [unwired: 1 in, 1 out]
        n227 = call <vilib>:"NT Read String Array.vi"("Name"="/TestMode/TestList") -> ("String Array"=w369:string[])  [unwired: 9 in, 1 out]
        n228 = Build Array (concatenate)("Select the test to run...", w369) -> (w368:string[])
        n229 = property on="Test Name" class="Ring (strict)"("Strings []"=w368) -> ()  [unwired: 2 in, 2 out]
      }
      event "Test Name": Value Change {
        w371 = FALSE ("Visible")
        # "Tell the robot the test name to run"
        n230 = event-data() -> ("NewVal"=w375:u16)  [unwired: 1 in]
        n231 = property on="Test Name" class="Ring (strict)"() -> ("Strings []"=w376:string[])  [unwired: 2 in, 2 out]
        n232 = local write "Progress"(T12 {"Test Progress"=0, "Test Progress Text"=""} ("Progress")) -> ()
        n233 = Index Array(array=w376, index=w375) -> (element=w374:string)
        n234 = call <vilib>:"NT Write String.vi"("String"=w374, "Name"="/TestMode/TestName") -> ()  [unwired: 9 in, 1 out]
        n235 = property on="Progress" class="Clust (strict)"("Visible"=TRUE) -> ()  [unwired: 2 in, 2 out]
        n236 = property on="Motor" class="Clust (strict)"("Visible"=w371) -> ()  [unwired: 2 in, 2 out]
        n237 = property on="Test Slider" class="Slide (strict)"("Visible"=w371) -> ()  [unwired: 2 in, 2 out]
        n238 = property on="On/Off" class="Bool (strict)"("Visible"=w371) -> ()  [unwired: 2 in, 2 out]
        n239 = property on="Rev/Fwd" class="Clust (strict)"("Visible"=w371) -> ()  [unwired: 2 in, 2 out]
        n240 = property on="Test Ring" class="Ring (strict)"("Visible"=w371) -> ()  [unwired: 2 in, 2 out]
      }
      event "Select Auto": Mouse Enter {
        # "Populate the combo box with the list of autonomous options"
        n241 = event-data() -> ()  [unwired: 1 in, 1 out]
        n242 = call <vilib>:"NT Read String Array.vi"("Name"="Auto List") -> ("String Array"=w378:string[])  [unwired: 9 in, 1 out]
        n243 = property on="Select Auto" class="CmbBox"("Strings[]"=w378) -> ()  [unwired: 2 in, 2 out]
      }
      event "Select Auto": Value Change {
        # "User modified the Auto Selection. Write to NT variable so robot knows."
        n244 = event-data() -> ("NewVal"=w381:string)  [unwired: 1 in]
        n245 = call <vilib>:"NT Write String.vi"("String"=w381, "Name"="Auto Selector") -> ()  [unwired: 9 in, 1 out]
      }
      event "Command Selection": Value Change {
        # "Get the params and show in table"
        n246 = event-data() -> ("NewVal"=w387:i32)  [unwired: 1 in]
        n247 = property on="Command Selection" class="MCListbox (strict)"() -> ("ItemNames"=w385:string[][])  [unwired: 2 in, 2 out]
        n248 = call <vilib>:"WPI_DashboardUpdate Command Params.vi"("NewVal"=w387, "Commands"=w385, "Param Tbl"=w386) -> ()  [unwired: 8 in, 1 out]
      }
      event "Execute Command": Value Change {
        # "Started one, Unique ID holds\nresponse"
        n249 = event-data() -> ()  [unwired: 1 in, 1 out]
        n250 = property on="Command Selection" class="MCListbox (strict)"() -> ("ItemNames"=w398:string[][])  [unwired: 2 in, 2 out]
        n251 = Index Array(array=w398, index (row)="Command Selection", index (col)=0) -> (element=w396:string)
        n252 = call <vilib>:"Invoke Commands.vi"("Command Params"="Command Params", "Function Name"=w396) -> ("Params"=w392:u8, "Started"=w391:bool)  [unwired: 7 in, 1 out]
        n253 = Array Subset(array="Command Params", length (row)=w392) -> (w393:string[][])  [unwired: 3 in]
        n254 = Select(t="Executing" ("Cmd Status"), s=w391, f="" ("Cmd Status")) -> (s? t:f=→"Cmd Status":string)
      }
      event "Command Selection": Double Click {
        n255 = event-data() -> ("Row"=w406:i32)  [unwired: 1 in]
        n256 = property on="Command Selection" class="MCListbox (strict)"() -> ("ItemNames"=w409:string[][])  [unwired: 2 in, 2 out]
        n257 = local read "Command Params"() -> (w405:string[][])
        n258 = Index Array(array=w409, index (row)=w406, index (col)=0) -> (element=w407:string)
        n259 = call <vilib>:"Invoke Commands.vi"("Command Params"=w405, "Function Name"=w407) -> ("Params"=w404:u8, "Started"=w399:bool)  [unwired: 7 in, 1 out]
        n260 = Array Subset(array=w405, length (row)=w404) -> (w403:string[][])  [unwired: 3 in]
        n261 = Select(t="Executing" ("Cmd Status"), s=w399, f="" ("Cmd Status")) -> (s? t:f=w400:string)
        n262 = local write "Cmd Status"(w400) -> ()
      }
      event "CheckList": Double Click {
        # "Shift clears all"
        # "Update symbols on the listbox"
        n263 = event-data() -> ("PlatMods.Shift"=w411:bool, "Row"=w413:i32)  [unwired: 1 in]
        n264 = case shown="True" w411 {
          tunnel: w413 -> [w417 _]
          tunnel: 1 -> [w416 _]
          frame False {
            n265 = property on="CheckList" class="LstBox (strict)"() -> ("Item Symbols"=w415:i32[])  [unwired: 2 in, 2 out]
            n266 = Replace Array Subset(array=w415, new element=w416, index=w417) -> (w414:i32[])
            n267 = property on="CheckList" class="LstBox (strict)"("Item Symbols"=w414) -> ()  [unwired: 2 in, 2 out]
          }
          frame True {
            w418 = 0 ("Top Row")
            n268 = property on="CheckList" class="LstBox (strict)"() -> ("Number of Rows"=w420:u32)  [unwired: 2 in, 2 out]
            n269 = Initialize Array(0, w420) -> (w419:i32[])
            n270 = property on="CheckList" class="LstBox (strict)"("Top Row"=w418, "Value"=w418, "Item Symbols"=w419) -> ()  [unwired: 2 in, 2 out]
          }
        }
      }
      event "CheckList": Key Down {
        # "Update symbols on the listbox\nLeft and right keys check and uncheck"
        n271 = event-data() -> ("VKey"=w424:T25)  [unwired: 1 in]
        n272 = case shown="\"Left\", \"Right\"" w424 {
          selector: w424 -> [w429 _]
          tunnel: eventvkey."Left" ("VKey") -> [w427 _]
          frame "Left", "Right" {
            n273 = Equal?(x=w427, y=w429) -> (x = y?=w428:bool)
            n274 = Select(t=0, s=w428, f=1) -> (s? t:f=w430:i32)
            n275 = property on="CheckList" class="LstBox (strict)"() -> ("Item Symbols"=w433:i32[])  [unwired: 2 in, 2 out]
            n276 = Replace Array Subset(array=w433, new element=w430, index="CheckList") -> (w432:i32[])
            n277 = property on="CheckList" class="LstBox (strict)"("Item Symbols"=w432) -> ()  [unwired: 2 in, 2 out]
          }
          frame Default {
          }
        }
      }
      event "Motor.Enable": Value Change {
        # "When the test mode otor enable helper is set, update that\ntree row item's value"
        n278 = event-data() -> ("NewVal"=w439:bool)  [unwired: 1 in]
        n279 = Unbundle("Motor") -> ("Value"=w438:dbl)  [unwired: 1 out]
        n280 = Select(t=w438, s=w439, f=0.0) -> (s? t:f=w436:dbl)
        n281 = call <vilib>:"NT Write Number.vi"("Numeric"=w436, "Name"=w435) -> ()  [unwired: 9 in, 1 out]
      }
      event "Test Slider": Value Change {
        # "When the test mode slider helper is set, update that\ntree row item's value"
        n282 = event-data() -> ("NewVal"=w442:dbl)  [unwired: 1 in]
        n283 = call <vilib>:"NT Write Number.vi"("Numeric"=w442, "Name"=w443) -> ()  [unwired: 9 in, 1 out]
      }
      event "On/Off": Value Change {
        # "When the test mode on/off helper value is set, update that\ntree row item's value"
        n284 = event-data() -> ("NewVal"=w447:bool)  [unwired: 1 in]
        n285 = Boolean To (0,1)(Boolean=w447) -> (0, 1=w446:i16)
        n286 = call <vilib>:"NT Write Number.vi"("Numeric"=w446, "Name"=w445) -> ()  [unwired: 9 in, 1 out]
      }
      event "Rev/Fwd": Value Change {
        # "When the test mode helper value for relays is set, update that\ntree row item's value"
        n287 = event-data() -> ("NewVal.Forward"=w455:bool, "NewVal.Reverse"=w454:bool)  [unwired: 1 in]
        n288 = Boolean To (0,1)(Boolean=w455) -> (0, 1=w451:i16)
        n289 = Boolean To (0,1)(Boolean=w454) -> (0, 1=w453:i16)
        n290 = Negate(x=w453) -> (-x=w452:i16)
        n291 = Add(x=w451, y=w452) -> (x+y=w450:i16)
        n292 = call <vilib>:"NT Write Number.vi"("Numeric"=w450, "Name"=w449) -> ()  [unwired: 9 in, 1 out]
      }
      event "Test Ring": Value Change {
        # "When a test mode helper value is selected from the ring,\nset the tree item's variable to the string value"
        n293 = event-data() -> ("NewVal"=w459:u16)  [unwired: 1 in]
        n294 = property on="Test Ring" class="Ring (strict)"() -> ("Strings []"=w460:string[])  [unwired: 2 in, 2 out]
        n295 = Index Array(array=w460, index=w459) -> (element=w458:string)
        n296 = call <vilib>:"NT Write String.vi"("String"=w458, "Name"=w457) -> ()  [unwired: 9 in, 1 out]
      }
      event "Rec Mode": Value Change {
        # "Update globals for recording mode and path to read log from.\nClear when logging and let NetworkTables set path for vision to\nuse."
        n297 = event-data() -> ("NewVal"=w471:enum32{"Stop", "Record", "Playback"})  [unwired: 1 in]
        n298 = global write "WPI_DashboardLogging Global.vi" "Logging Filename"(path "") -> ()
        n299 = global write "WPI_DashboardLogging Global.vi" "Recording"(w471) -> ()
        n300 = case shown="\"Playback\"" w471 {
          tunnel: w470 -> [_ w473 w482]
          tunnel: [_ _ w481] -> w468
          tunnel: [_ _ w480] -> _
          tunnel: w466 -> [_ _ w478]
          tunnel: cluster{i32, i32} {-250, 170} -> [_ _ w477]
          tunnel: [_ _ T26 {"Image Size"=TRUE, "Image Type"=TRUE, "Pixel Value"=TRUE, "ROI Information"=TRUE, "Zoom Factor"=FALSE} ("Image Information Shown:All Elements")] -> w464
          tunnel: [_ _ TRUE ("Zoom Factor")] -> w463
          tunnel: w462 -> [_ _ w474]
          frame Default {
          }
          frame "Stop", "Record" {
            # "Place Window too"
            n301 = invoke class="VI" method="FP.Close"(reference=w473) -> (reference out=w472:refnum<vi>)  [unwired: 2 in, 2 out]
            n302 = invoke class="VI" method="Abort VI"(reference=w472) -> ()  [unwired: 2 in, 3 out]
          }
          frame "Playback" {
            n303 = call "Open Playback Panel.vi"("Offset"=w477, "DB VI Ref"=w478, "Playback in"=w482) -> ("Playback out"=w479:refnum<vi>)  [unwired: 8 in]
            n304 = register-events(w479, w474) -> (reference out=w481:refnum<event-registration>, error out=w480:errorcluster)  [unwired: 2 in]
          }
        }
        n305 = property on="Camera Image" class="ImageControl"("Image Information Shown"=w464, "Image Information Visible"=w463) -> ()  [unwired: 2 in, 2 out]
        n306 = call <vilib>:"WPI_DashboardNT Log FieldName Cache.vi"("Operation"=enum16{"Lookup/Add", "Index", "Clear"}."Clear") -> ()  [unwired: 8 in, 3 out]
      }
      event Panel Close {
        w484 = enum32{"Stop", "Record", "Playback"}."Stop" ("Rec Mode")
        # "Playback window has been closed, abort"
        n307 = event-data() -> ()  [unwired: 1 in, 4 out]
        n308 = local write "Rec Mode"(w484) -> ()
        n309 = global write "WPI_DashboardLogging Global.vi" "Recording"(w484) -> ()
      }
      event Panel Close {
        # "Abort playback window and ourself"
        n310 = event-data() -> ()  [unwired: 1 in, 4 out]
        n311 = invoke class="VI" method="FP.Close"(reference=w488) -> (reference out=w487:refnum<vi>)  [unwired: 2 in, 2 out]
        n312 = invoke class="VI" method="Abort VI"(reference=w487) -> (error out=w486:errorcluster)  [unwired: 2 in, 2 out]
        n313 = invoke class="VI" method="Abort VI"(error in=w486) -> ()  [unwired: 2 in, 3 out]
      }
      event User Event {
        n314 = event-data() -> ("IDs"=w495:cluster{"RPC field ID":u16, "Unique ID":u16}, "String"=w494:string)  [unwired: 1 in]
        n315 = Bundle("IDs"=w495, "String"=w494) -> (w493:T14)  [unwired: 1 in]
        n316 = call <vilib>:"Retrieve RPC Response.vi"("RPC Response"=w493) -> ("Output"=w491:string[][])  [unwired: 10 in]
        n317 = Build Array (concatenate)(w489, w491) -> (w490:string[][])
        n318 = local write "Command Params"(w490) -> ()
        n319 = local write "Cmd Status"("" ("Cmd Status")) -> ()
      }
      event "Tree": Double Click {
        n320 = event-data() -> ("PlatMods"=w499:T29, "Tag"=w498:string)  [unwired: 1 in]
        n321 = Unbundle(w499) -> ("Shift"=w497:bool)  [unwired: 4 out]
        n322 = Not(x=w497) -> (.not. x?=w496:bool)
        n323 = call <vilib>:"NT Update Persistence.vi"("Persistence"=w496, "Name"=w498) -> ()  [unwired: 9 in, 1 out]
      }
    }
  }
  n324 = while {
    tunnel: w64 -> [w502]
    i -> [w505]
    stop <- FALSE stop-if-true
    n325 = Wait (ms)(milliseconds to wait=u32 100) -> ()  [unwired: 1 out]
    n326 = case shown="\"Playback\"" "Rec Mode" {
      tunnel: w505 -> [_ _ w520]
      tunnel: [u32 2829099 ("Base Color") u32 11141120 ("Target Color") w509] -> w501
      frame "Stop", Default {
        # "Reset the color, extra updates don't cost much"
      }
      frame "Record" {
      }
      frame "Playback" {
        # "Playback"
        n327 = Quotient & Remainder(x=w520, y=u32 50 ("milliseconds to wait")) -> (x-y*floor(x/y)=w516:u32)  [unwired: 1 out]
        n328 = Divide(x=w516, y=u32 50 ("milliseconds to wait")) -> (x/y=w513:dbl)
        n329 = Multiply(x=6.283185307179586, y=w513) -> (x*y=w518:dbl)
        n330 = Sine(x=w518) -> (sin(x)=w517:dbl)
        n331 = Absolute Value(x=w517) -> (abs(x)=w510:dbl)
        n332 = call "Interpolate RGB Color.vi"("Proportion"=w510, "Target Color"=u32 30976, "Base Color"=u32 2829099) -> ("Result Color"=w509:u32)  [unwired: 8 in]
      }
    }
    n333 = property class="Pane"(reference=w502, "PaneColor"=w501) -> ()  [unwired: 1 in, 2 out]
  }
  n334 = local write "Dashboard Tab"(T2."Drive" ("Dashboard Tab")) -> ()
  n335 = property on="On/Off" class="Bool (strict)"("Visible"=w34) -> ()  [unwired: 2 in, 2 out]
  n336 = property on="Motor" class="Clust (strict)"("Visible"=w34) -> ()  [unwired: 2 in, 2 out]
  n337 = property on="Progress" class="Clust (strict)"("Visible"=w34) -> ()  [unwired: 2 in, 2 out]
  n338 = property on="Test Ring" class="Ring (strict)"("Visible"=w34) -> ()  [unwired: 2 in, 2 out]
  n339 = property on="Rev/Fwd" class="Clust (strict)"("Visible"=w34) -> ()  [unwired: 2 in, 2 out]
  n340 = local write "Command Selection"(u16 0 ("milliseconds to wait")) -> ()
  n341 = local write "Command Params"(string[][] [] ("Command Params")) -> ()
  n342 = global write "WPI_DashboardLogging Global.vi" "Recording"(w58) -> ()
  n343 = local write "Rec Mode"(w58) -> ()
  n344 = while {
    tunnel: u16 1741 ("timeout ms (25000)") -> [w522]
    stop <- FALSE stop-if-true
    n345 = TCP Create Listener(10:w522) -> (0:w521:errorcluster, 3:w523:refnum<k5>)  [unwired: 4 in, 1 out]
    n346 = case shown="No Error" w521 {
      selector: w521 -> [w525 _]
      tunnel: w523 -> [w526 _]
      frame No Error {
        n347 = while {
          tunnel: w526 -> [w529]
          tunnel: w525 -> [w528]
          stop <- FALSE stop-if-true
          n348 = TCP Wait On Listener(8:w528, 11:w529) -> (0:w530:errorcluster, 4:w531:refnum<k5>)  [unwired: 2 in, 3 out]
          n349 = local write "TCP"(w531) -> ()
          n350 = case shown="No Error" w530 {
            frame No Error {
            }
            frame Error {
              n351 = Wait (ms)(milliseconds to wait=u32 1000) -> ()  [unwired: 1 out]
            }
          }
        }
      }
      frame Error {
        n352 = Wait (ms)(milliseconds to wait=u32 1000) -> ()  [unwired: 1 out]
      }
    }
  }
  n353 = call <vilib>:"NT Write String.vi"("String"="Select Auto", "Name"="Auto Selector") -> ()  [unwired: 9 in, 1 out]
